vi "Write Voltage2.vi"(8 "error in (no error)":errorcluster, 9 "Current voltage":dbl, 10 "Desired voltage":dbl, 11 "Refnum in":refnum<k21>) -> (0 "error out":errorcluster, 3 "Refnum out":refnum<k21>)   [LabVIEW 2018]
uses:
  <vilib>/Analysis/NI_AALBase.lvlib
  <vilib>/Analysis/1siggen.llb/Ramp Pattern by Samples.vi
  Samples per channle (Generation) - Global Variable.vi
  <vilib>/DAQmx/write.llb/DAQmx Write (Analog 1D DBL 1Chan NSamp).vi
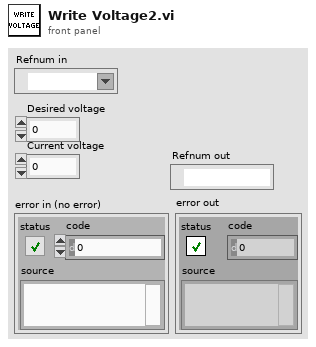
[diagram p1: front panel]
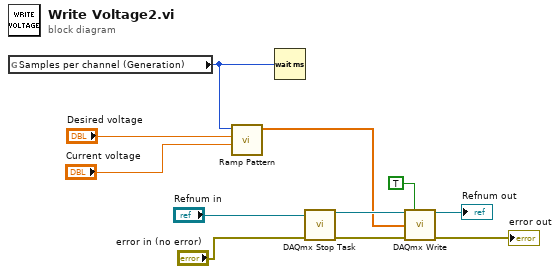
[diagram p0: block diagram]
diagram:
  n1 = global read "Samples per channle (Generation) - Global Variable.vi" "Samples per channel (Generation)"() -> (w1:i32)
  n2 = call-poly <vilib>:"Ramp Pattern.vi"("start"="Current voltage", "end"="Desired voltage", "samples"=w1) -> ("Ramp Pattern"=w2:dbl[])  [unwired: 7 in, 1 out]
  n3 = Wait (ms)(milliseconds to wait=w1) -> ()  [unwired: 1 out]
  n4 = call <vilib>:"DAQmx Stop Task.vi"("task/channels in"="Refnum in", "error in"="error in (no error)") -> ("task out"=w6:refnum<k21>, "error out"=w7:errorcluster)  [unwired: 12 in]
  n5 = call-poly <vilib>:"DAQmx Write.vi"("task/channels in"=w6, "auto start"=TRUE, "data"=w2, "error in"=w7) -> ("task out"=→"Refnum out":refnum<k21>, "error out"=→"error out":errorcluster)  [unwired: 9 in, 1 out]
